vi "INITIALIZE FUNCTION.vi"(8 "Error In Cluster":T3={"Unhandled Error"=FALSE, "Error"={"status"=FALSE, "code"=0, "source"=""}, "Message Type"=enum."Code", "Number of Values"=0, "Msg Value Type"=[], "Msg Ints"=[], "Msg Real Values"=[], "Msg String Values"=[], "Severity (Emergency)"=enum."Emergency"} {"Msg Real Values" format="%.2f"}, 10 "Tags":T1[](array[typedef]), 11 "Source":refnum<class "Source.lvclass">) -> (0 "Error Out Cluster":T2={"Unhandled Error"=FALSE, "Error"={"status"=FALSE, "code"=0, "source"=""}, "Message Type"=enum."Code", "Number of Values"=0, "Msg Value Type"=[], "Msg Ints"=[], "Msg Real Values"=[], "Msg String Values"=[], "Severity (Emergency)"=enum."Emergency"} {"Msg Real Values" format="%.2f"}, 2 "Tags out":T1[](array[typedef]), 3 "Source out":refnum<class "Source.lvclass">)   [LabVIEW 2013, in "Customer.TestSLATE.Mnemonic.lvlib"]
uses:
  Customer.TestSLATE.Mnemonic.lvlib
  <vilib>/Test SLATE/CLASSES/SOURCE/Source.lvclass
  <vilib>/Test SLATE/CONTROLS/Error In Cluster.ctl
  <vilib>/Test SLATE/CVT/Tag Information.ctl
  <vilib>/Test SLATE/CLASSES/TAG/TS_Tag.lvclass
  <vilib>/Test SLATE/CONTROLS/Error Out Cluster.ctl
  <vilib>/Test SLATE/Test SLATE.lvlib
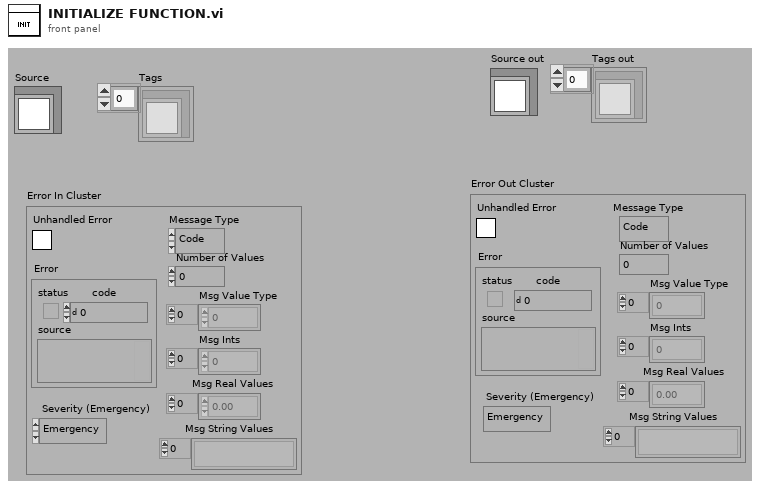
[diagram p1: front panel]
types:
  T1 = typedef "Test SLATE.lvlib/Tag Information.ctl" = refnum<class "TS_Tag.lvclass">
  T2 = typedef "Test SLATE.lvlib/Error Out Cluster.ctl" = cluster{"Unhandled Error":bool, "Error":errorcluster, "Message Type":enum8{"Code", "Text"}, "Number of Values":i8, "Msg Value Type":i32[], "Msg Ints":i32[], "Msg Real Values":sgl[], "Msg String Values":string[], "Severity (Emergency)":enum32{"Information", "Warning", "Emergency"}}
  T3 = typedef "Test SLATE.lvlib/Error In Cluster.ctl" = cluster{"Unhandled Error":bool, "Error":errorcluster, "Message Type":enum8{"Code", "Text"}, "Number of Values":i8, "Msg Value Type":i32[], "Msg Ints":i32[], "Msg Real Values":sgl[], "Msg String Values":string[], "Severity (Emergency)":enum32{"Information", "Warning", "Emergency"}}
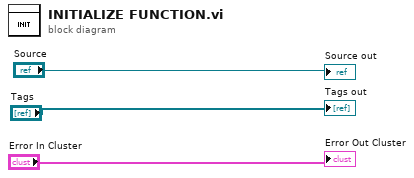
[diagram p0: block diagram]
diagram:
  "Source out" <- "Source"
  "Tags out" <- "Tags"
  "Error Out Cluster" <- "Error In Cluster"
